vi "arduino_commands.vi"(0 "Shutter off":bool, 1 "Shutter on":bool, 2 "Go to step":bool, 3 "Constant speed":bool, 4 "Current Step":bool, 5 "Set zero":bool, 6 "wait until completion? (T)":bool=TRUE, 8 "Stop":bool, 9 "Argumento":string, 10 "Número de motor":string, 11 "Directorio scripts ArduinoStepper.py":path=path "C:/Users/franjas/Documents/rutinas-calibracion-slm") -> (7 "Array":string[](array[string]))   [LabVIEW 2013]
uses:
  <vilib>/regexp/Match Regular Expression.xnode
panel:
  out "standard output":string
  in  "Set speed":bool
  in  "Comando":string
  out "Comando que está siendo enviado a python":string
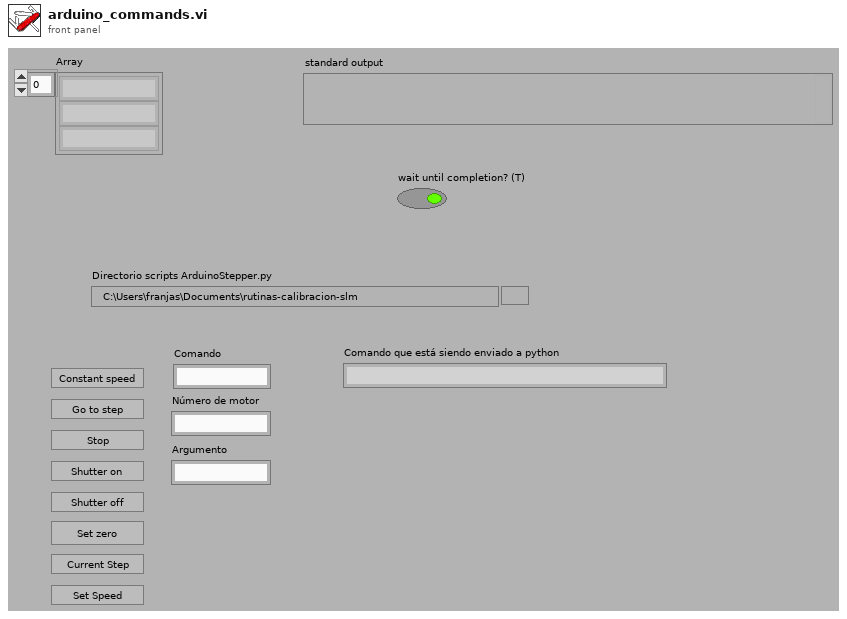
[diagram p1: front panel]
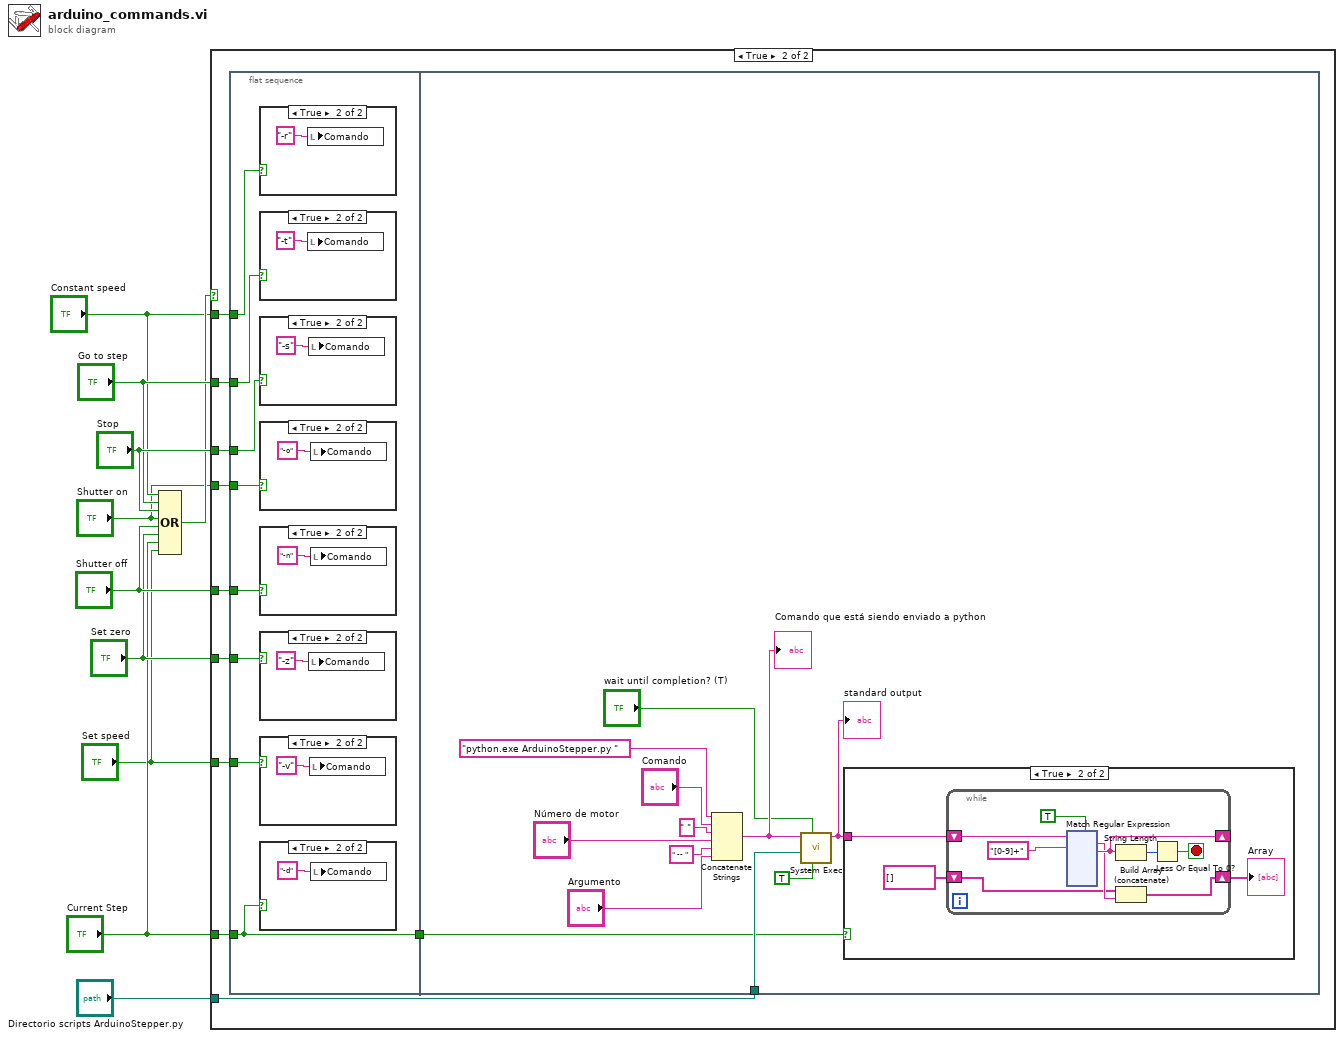
[diagram p0: block diagram]
diagram:
  n1 = Compound Arithmetic op=OR("Constant speed", "Go to step", "Stop", "Shutter on", "Shutter off", "Set zero", "Current Step", "Set speed") -> (w7:bool)
  n2 = case shown="True" w7 {
    tunnel: "Directorio scripts ArduinoStepper.py" -> [_ w18]
    tunnel: "Constant speed" -> [_ w20]
    tunnel: "Go to step" -> [_ w17]
    tunnel: "Stop" -> [_ w19]
    tunnel: "Shutter on" -> [_ w16]
    tunnel: "Shutter off" -> [_ w15]
    tunnel: "Set zero" -> [_ w14]
    tunnel: "Current Step" -> [_ w13]
    tunnel: "Set speed" -> [_ w11]
    frame False {
    }
    frame True {
      n3 = flat-sequence {
        tunnel: w20 -> [w28]
        tunnel: w17 -> [w27]
        tunnel: w19 -> [w26]
        tunnel: w16 -> [w25]
        tunnel: w15 -> [w24]
        tunnel: w14 -> [w23]
        tunnel: w13 -> [w22]
        tunnel: [w22] -> w12
        tunnel: w11 -> [w21]
        tunnel: w18 -> [w48]
        tunnel: w12 -> [w39]
        frame #0 {
          n4 = case shown="True" w28 {
            frame False {
            }
            frame True {
              n5 = local write "Comando"("-r" ("Comando")) -> ()
            }
          }
          n6 = case shown="True" w27 {
            frame False {
            }
            frame True {
              n7 = local write "Comando"("-t" ("Comando")) -> ()
            }
          }
          n8 = case shown="True" w26 {
            frame False {
            }
            frame True {
              n9 = local write "Comando"("-s" ("Comando")) -> ()
            }
          }
          n10 = case shown="True" w25 {
            frame False {
            }
            frame True {
              n11 = local write "Comando"("-o" ("Comando")) -> ()
            }
          }
          n12 = case shown="True" w24 {
            frame False {
            }
            frame True {
              n13 = local write "Comando"("-n" ("Comando")) -> ()
            }
          }
          n14 = case shown="True" w23 {
            frame False {
            }
            frame True {
              n15 = local write "Comando"("-z" ("Comando")) -> ()
            }
          }
          n16 = case shown="True" w21 {
            frame False {
            }
            frame True {
              n17 = local write "Comando"("-v" ("Comando")) -> ()
            }
          }
          n18 = case shown="True" w22 {
            frame False {
            }
            frame True {
              n19 = local write "Comando"("-d" ("Comando")) -> ()
            }
          }
        }
        frame #1 {
          n20 = Concatenate Strings("python.exe ArduinoStepper.py ", "Comando", " " ("string"), "Número de motor", " -- ", "Argumento") -> (w44:string)
          "Comando que está siendo enviado a python" <- w44
          n21 = call <vilib>:"System Exec.vi"("run minimized? (F)"=TRUE, "wait until completion? (T)"="wait until completion? (T)", "working directory"=w48, "command line"=w44) -> ("standard output"=w40:string)  [unwired: 4 in, 3 out]
          "standard output" <- w40
          n22 = case shown="True" w39 {
            tunnel: w40 -> [_ w51]
            frame False {
            }
            frame True {
              n23 = while {
                shift-right: [w58] -> _
                shift-left: w51 -> [w59]
                shift-right: [w55] -> w50
                shift-left: string[] [] -> [w53]
                stop <- w56 stop-if-true
                n24 = xnode "Match Regular Expression"("input string"=w59, "regular expression"="[0-9]+", "multiline? (F)"=TRUE) -> ("whole match"=w54:string, "after match"=w58:string)  [unwired: 3 in, 5 out]
                n25 = String Length(string=w58) -> (length=w57:i32)
                n26 = Build Array (concatenate)(w53, w54) -> (w55:string[])
                n27 = Less Or Equal To 0?(x=w57) -> (x <= 0?=w56:bool)
              }
              "Array" <- w50
            }
          }
        }
      }
    }
  }
